vi "Main.vi"() -> ()   [LabVIEW 2020]
uses:
  <vilib>/userDefined/High Color/IMAQdx.ctl
  <vilib>/vision/Image Controls.llb/IMAQ Image.ctl
  <vilib>/DAQmx/read.llb/DAQmx Read (Analog Wfm 1Chan NSamp).vi
  <vilib>/Utility/error.llb/Error Cluster From Error Code.vi
  <vilib>/DAQmx/miscellaneous.llb/DAQmx Fill In Error Info.vi
  <vilib>/ErrorRing/Error Ring.xnode
  SuportVI2/Message Queue/Message Queue.lvlib
  SuportVI2/User Event - Stop/User Event - Stop.lvlib
  <vilib>/vision/driver/NI_Vision_Acquisition_Software.lvlib
panel:
  in  "Is start 2":bool=TRUE
  in  "Data":string="000001"
  in  "Is start":bool
  out "Waveform Graph":waveform(dbl)(graph)
  in  "Aquire Configuration":T1
  in  "Generator Configuration":T1
  out "Image":T2(plugin-control)
  in  "Camera Config":cluster{"Camera Select":T3}={"Camera Select"="cam0"}
  in  "Exit":bool
  in  "Stop Camera":bool
  in  "Start":bool
  out "Status Line":string
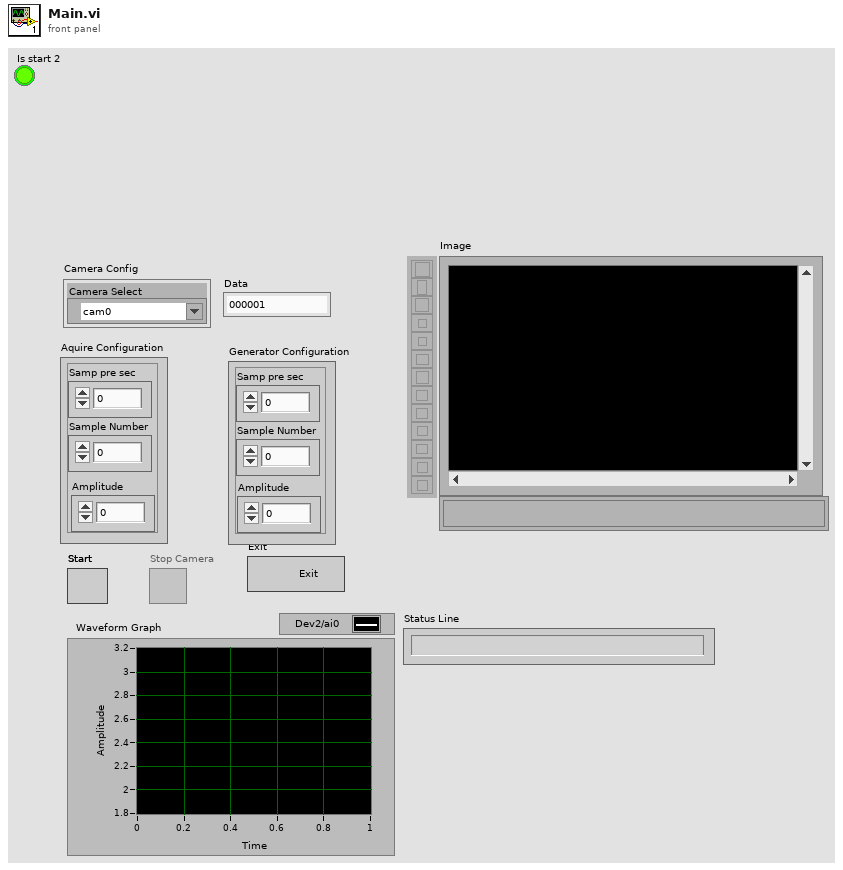
[diagram p1: front panel]
types:
  T1 = cluster{"Sample Number":dbl, "Samp pre sec":i32, "Amplitude":dbl}
  T2 = typedef "IMAQ Image.ctl" = refnum<image>
  T3 = typedef "IMAQdx.ctl" = refnum<k21>
  T4 = cluster{"configuration file path out":path, "DAQmx Task":refnum<k21>, "DAQmx Chanel":cluster{"SampClk.Rate":dbl, "SampQuant.SampPerChan":i32, "Amplitude 2":dbl}}
  T5 = cluster{"DAQmx Task":refnum<k21>, "DB Data":dbl[][], "DAQmx Chanel":cluster{"SampClk.Rate":dbl, "SampQuant.SampPerChan":i32, "Amplitude":dbl}}
  T6 = cluster{"Image":cluster{"Image original":T2, "Image copy":T2, "Image Out":T2}, "Session Config":cluster{"Session":T3}, "Data":string}
  T7 = cluster{"Start Camera":refnum<vi>, "Stop Camera":refnum<vi>, "Exit":refnum<vi>, "Camera Conf":refnum<vi>, "Status Line":refnum<vi>, "Status Line Text":string, "Camera Select":refnum<vi>, "Start Acquire":refnum<vi>, "Stop Acquire":refnum<vi>, "Start SinusGen":refnum<vi>, "Stop SinusGen":refnum<vi>, "Generator Configuration":refnum<vi>, "Aquire Configuration":refnum<vi>}
  T8 = cluster{"UI":refnum<queue>, "Camera":refnum<queue>, "Acquire":refnum<queue>, "SinusGen":refnum<queue>}
  T9 = typedef "Image Type" = u32
  T10 = cluster{"SampClk.Rate":dbl, "SampQuant.SampPerChan":i32, dbl}
  T11 = cluster{"SampClk.Rate":dbl, "SampQuant.SampPerChan":i32, "Amplitude":dbl}
  T12 = cluster{"SampClk.Rate":dbl, "SampQuant.SampPerChan":i32, "Amplitude 2":dbl}
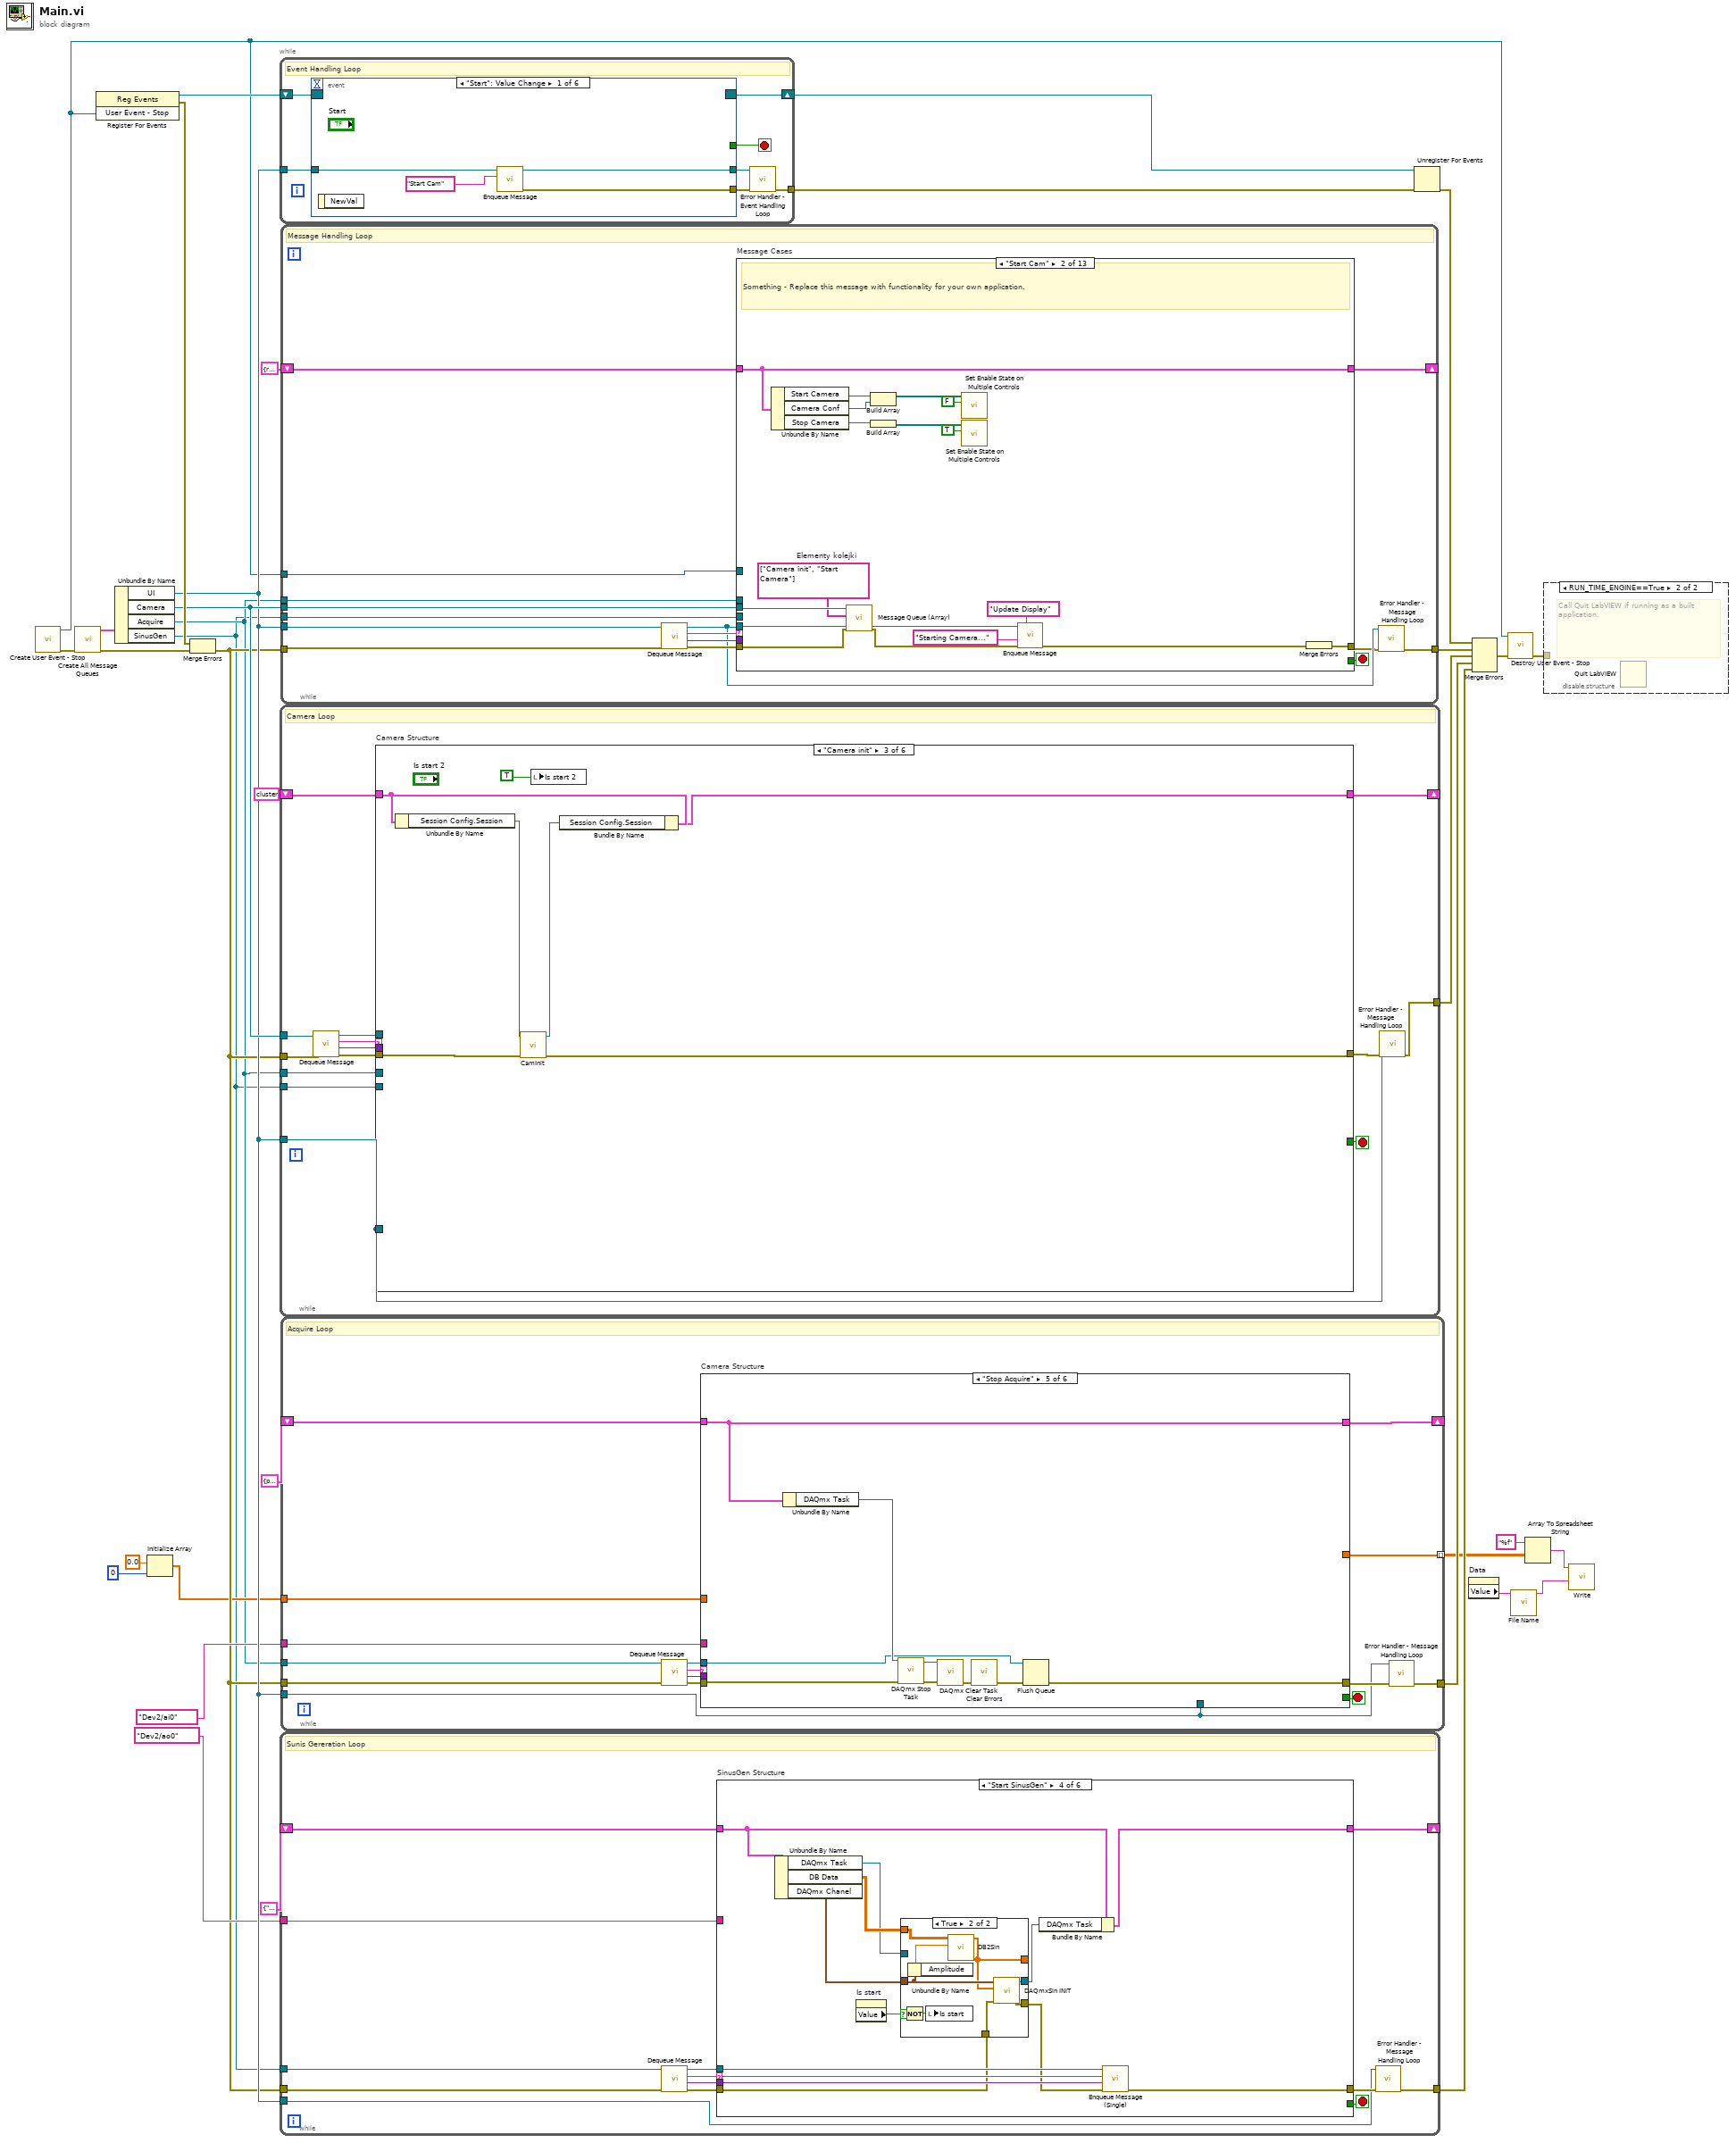
[diagram p0: block diagram]
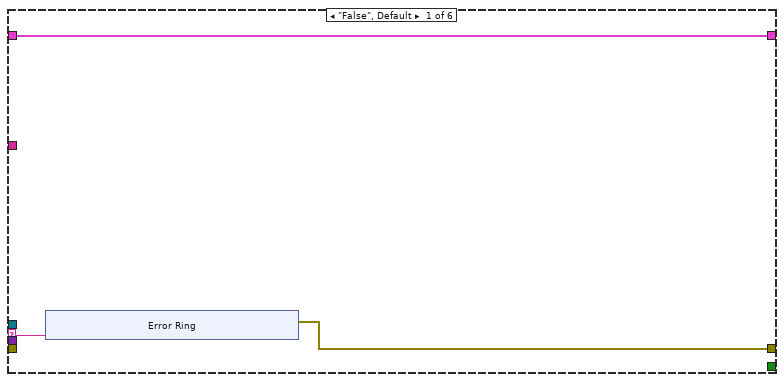
[diagram p2: hidden frame]
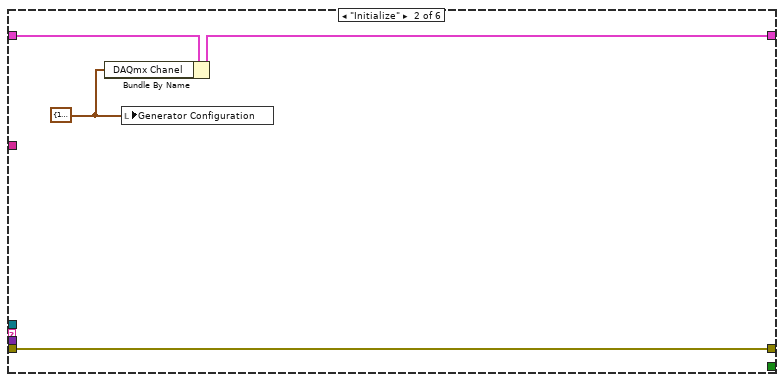
[diagram p3: hidden frame]
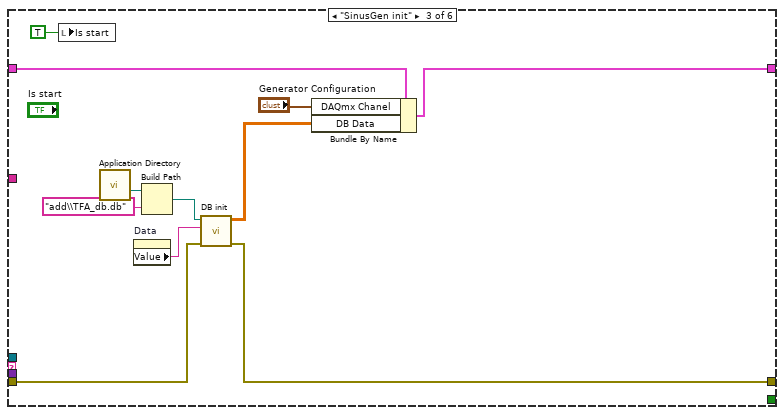
[diagram p4: hidden frame]
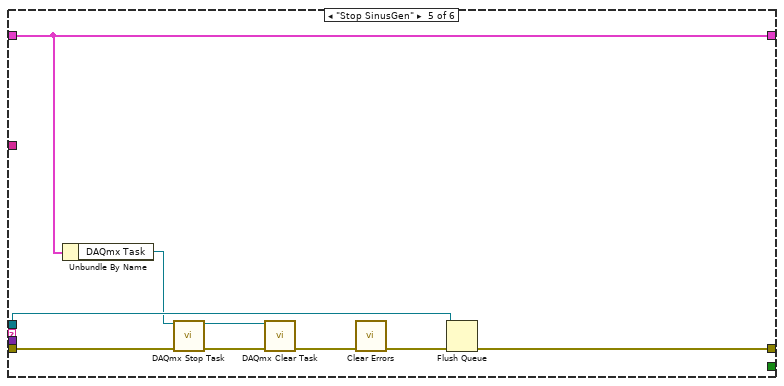
[diagram p6: hidden frame]
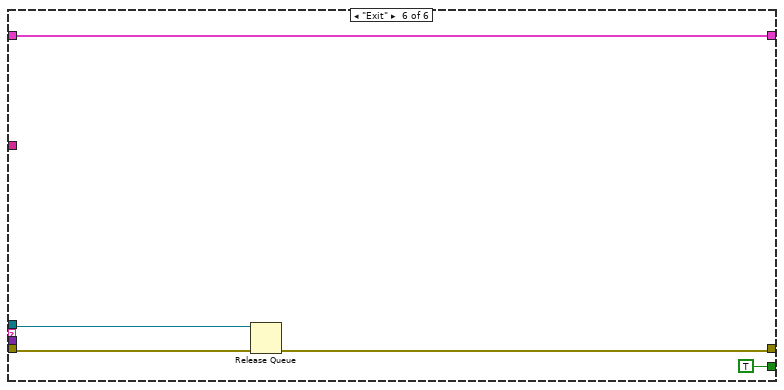
[diagram p7: hidden frame]
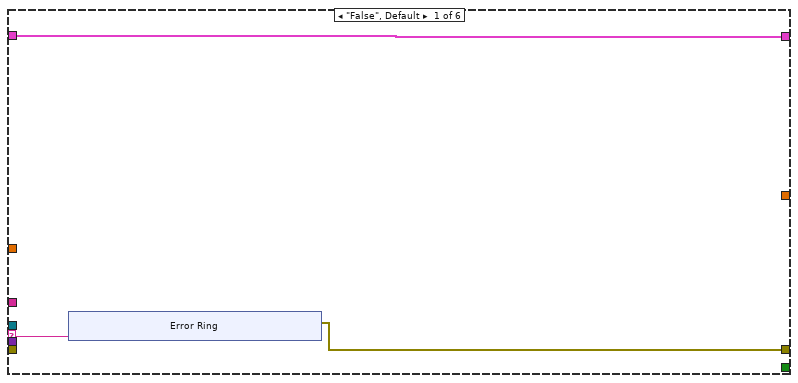
[diagram p8: hidden frame]
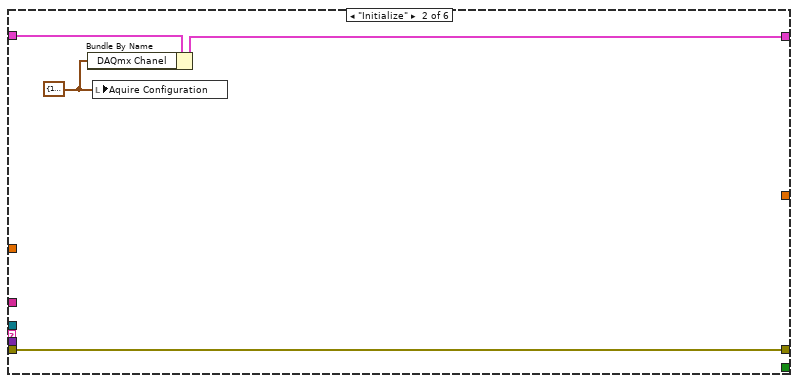
[diagram p9: hidden frame]
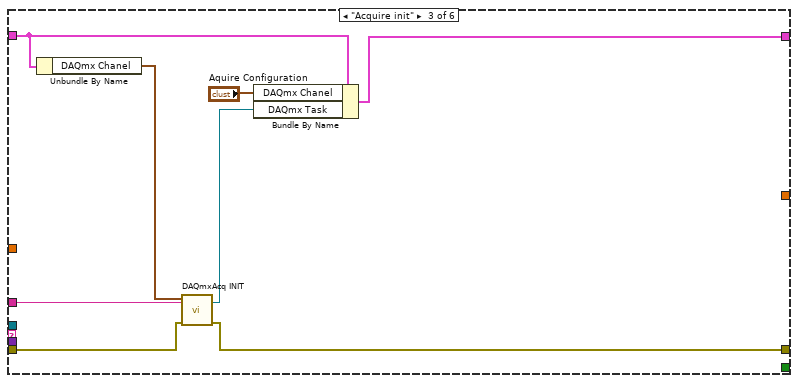
[diagram p10: hidden frame]
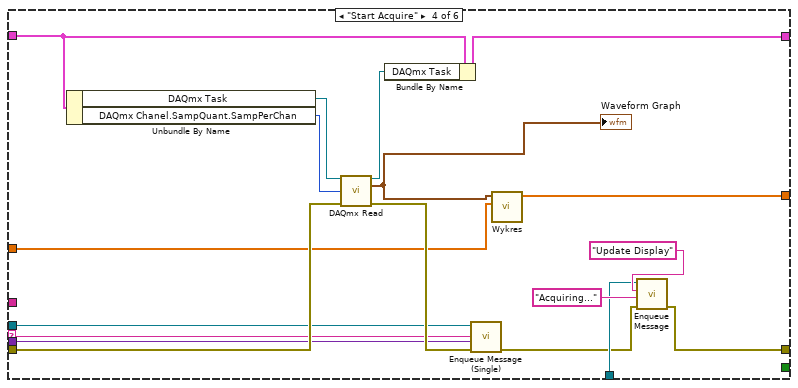
[diagram p11: hidden frame]
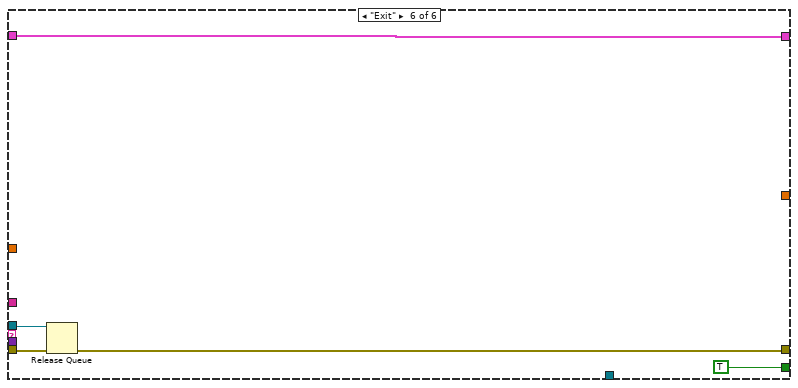
[diagram p12: hidden frame]
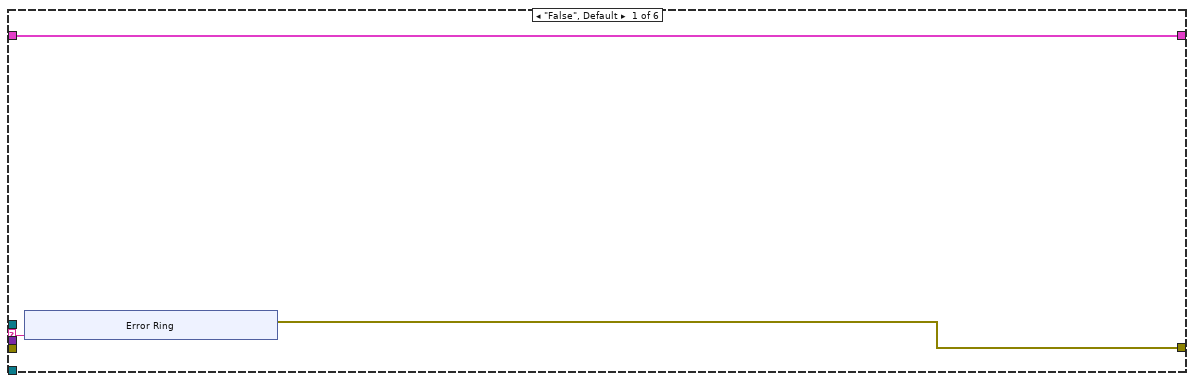
[diagram p13: hidden frame]
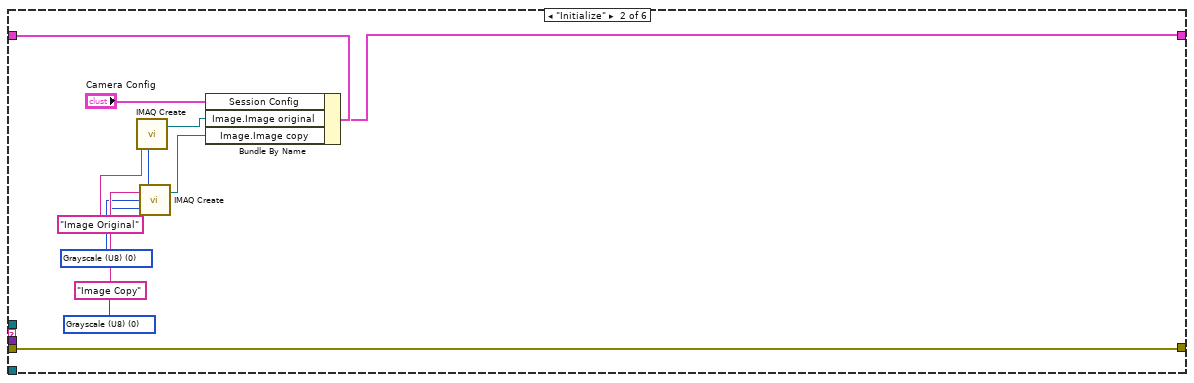
[diagram p14: hidden frame]
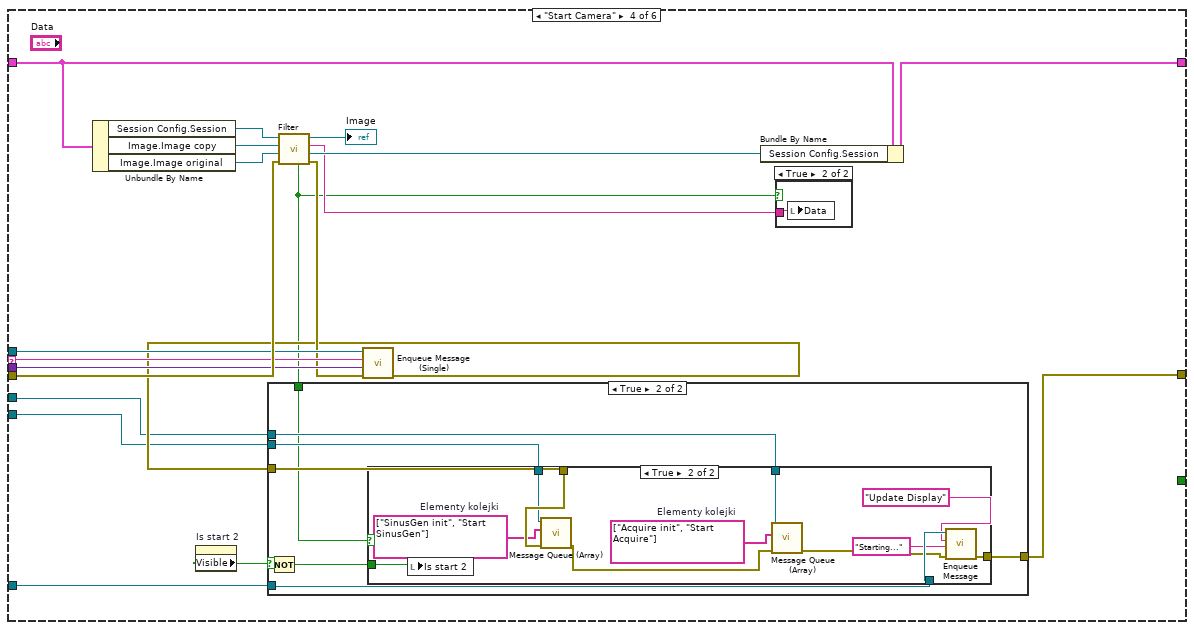
[diagram p15: hidden frame]
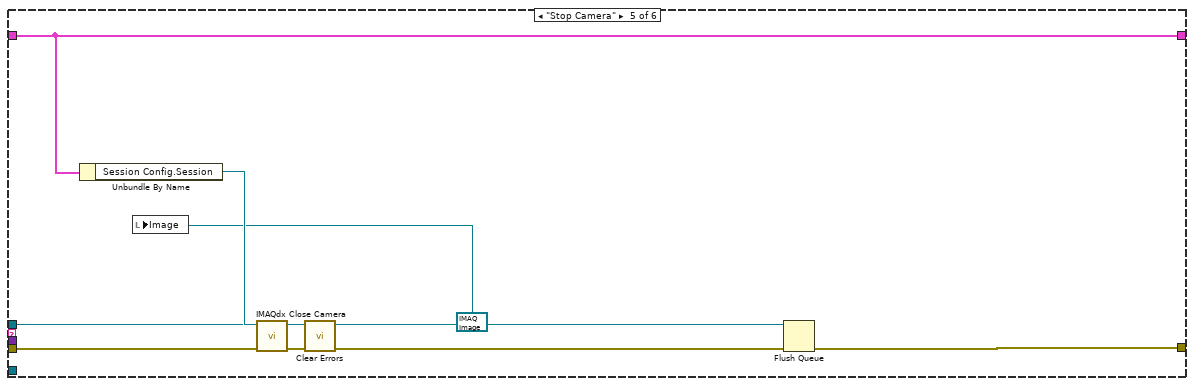
[diagram p19: hidden frame]
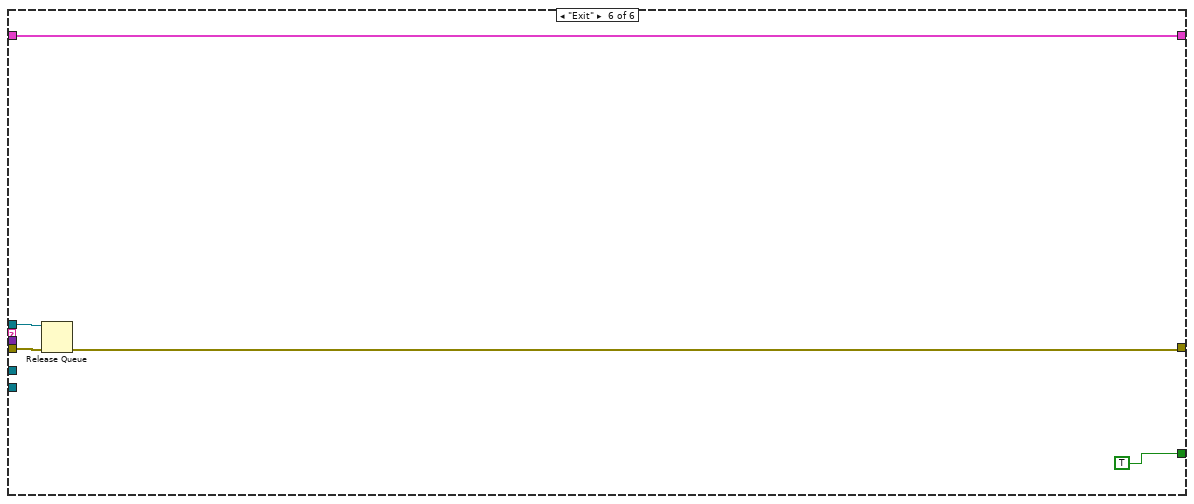
[diagram p20: hidden frame]
diagram:
  n1 = call "Create User Event - Stop.vi"() -> ("error out"=w32:errorcluster, "User Event - Stop"=w18:refnum<user-event>)  [unwired: 10 in]
  n2 = call "Create All Message Queues.vi"("error in (no error)"=w32) -> ("error out"=w34:errorcluster, "Message Queues out"=w22:T8)  [unwired: 9 in]
  n3 = register-events(w18) -> (reference out=w27:refnum<event-registration>, error out=w26:errorcluster)  [unwired: 2 in]
  n4 = Unbundle By Name(w22) -> ("UI"=w20:refnum<queue>, "Camera"=w21:refnum<queue>, "Acquire"=w2:refnum<queue>, "SinusGen"=w1:refnum<queue>)
  n5 = Initialize Array(0.0 ("element"), 0 ("dimension size")) -> (w6:dbl[])
  n6 = Merge Errors(w26, w34) -> (w14:errorcluster)
  n7 = while {
    tunnel: w20 -> [w41]
    shift-right: [w39] -> w30
    shift-left: w27 -> [w40]
    tunnel: [w35] -> w28
    stop <- w37 stop-if-true
    # "Event Handling Loop"
    n8 = event shown="[0] \"Start\": Value Change" {
      selector: w40 -> [_ _ _ _ _ _]
      dyn-events: [_ _ _ _ _ _] -> w39
      timeout: _ -> [_ _ _ _ _ _]
      tunnel: [_ _ _ _ _ TRUE ("Discard?")] -> w37
      tunnel: w41 -> [w45 w49 w54 w56 w61 w64]
      tunnel: [w42 w46 w53 _ w60 _] -> w38
      tunnel: [w44 w48 w52 w56 w59 w64] -> w36
      event "Start": Value Change {
        n9 = event-data() -> ()  [unwired: 1 in, 1 out]
        n10 = call-poly "Enqueue Message.vi"("Message"="Start Cam", "Message Queue"=w45) -> ("error out"=w42:errorcluster, "dup Message Queue"=w44:refnum<queue>)  [unwired: 8 in]
      }
      event "Stop Camera": Value Change {
        n11 = event-data() -> ()  [unwired: 1 in, 1 out]
        n12 = call-poly "Enqueue Message.vi"("Message"="Stop Cam", "Message Queue"=w49) -> ("error out"=w46:errorcluster, "dup Message Queue"=w48:refnum<queue>)  [unwired: 8 in]
      }
      event Panel Close? {
        # "Send the 'Confirm Quit' message if the user closes the panel of the VI. Discard the event so the 'Confirm Quit' message has a chance to run."
        n13 = event-data() -> ()  [unwired: 1 in, 1 out]
        n14 = call-poly "Enqueue Message.vi"("Priority Message? (F)"=TRUE, "Message"="Confirm Quit", "Message Queue"=w54) -> ("error out"=w53:errorcluster, "dup Message Queue"=w52:refnum<queue>)  [unwired: 7 in]
        n15 = event-data("Discard?"=TRUE) -> ()  [unwired: 1 in, 1 out]
      }
      event Application Instance Close {
        # "#CodeRecommended - When a project closes, all VIs within that project are aborted and leave memory. However, any code placed in this event frame is guaranteed to run to completion, so add any cleanup code that absolutely must happen here."
        n16 = event-data() -> ()  [unwired: 1 in, 1 out]
      }
      event "Exit": Value Change {
        n17 = event-data() -> ()  [unwired: 1 in, 1 out]
        n18 = call-poly "Enqueue Message.vi"("Priority Message? (F)"=TRUE, "Message"="Exit", "Message Queue"=w61) -> ("error out"=w60:errorcluster, "dup Message Queue"=w59:refnum<queue>)  [unwired: 7 in]
      }
      event User Event {
        # "The Message Handling Loop processed an \"Exit\" message, which fired this event to stop the Event Handling Loop."
        n19 = event-data() -> ()  [unwired: 1 in, 1 out]
        n20 = local write "Status Line"("Exiting application" ("VI Stopped")) -> ()
      }
    }
    n21 = call "Error Handler - Event Handling Loop.vi"("error in (no error)"=w38, "Message Queue"=w36) -> ("dup error in"=w35:errorcluster)  [unwired: 8 in, 1 out]
  }
  n22 = while {
    shift-right: [w71] -> _
    shift-left: T6 {"Image"={"Image original"=refnum, "Image copy"=refnum, "Image Out"=refnum}, "Session Config"={"Session"=""}, "Data"=""} ("Camera conf Cluster") -> [w74]
    tunnel: [w78] -> w24
    tunnel: w14 -> [w77]
    tunnel: w20 -> [w65]
    tunnel: w21 -> [w73]
    tunnel: w2 -> [w67]
    tunnel: w1 -> [w66]
    stop <- w69 stop-if-true
    # "Camera Loop"
    n23 = call "Dequeue Message.vi"("error in (no error)"=w77, "Message Queue"=w73) -> ("error out"=w76:errorcluster, "Message Data"=w70:variant, "Message"=w68:string, "dup Message Queue"=w72:refnum<queue>)  [unwired: 6 in]
    n24 = case "Camera Structure" shown="\"Camera init\"" w68 {
      selector: w68 -> [w79 _ _ w117 _ _]
      tunnel: [w81 w98 w102 w109 w151 w159] -> w75
      tunnel: w76 -> [_ w98 w103 w125 w156 w158]
      tunnel: w74 -> [w80 w96 w101 w121 w155 w161]
      tunnel: w72 -> [_ _ _ w118 w150 w160]
      tunnel: [w80 w95 w100 w119 w155 w161] -> w71
      tunnel: w70 -> [_ _ _ w116 _ _]
      tunnel: [_ _ _ _ _ TRUE] -> w69
      tunnel: w67 -> [_ _ _ w106 _ _]
      tunnel: w66 -> [_ _ _ w110 _ _]
      tunnel: w65 -> [_ _ _ w112 _ _]
      frame "False", Default {
        n25 = xnode "Error Ring"("parameter 0"=w79) -> ("error out"=w81:errorcluster)
      }
      frame "Initialize" {
        w90 = T9 0 items=["Grayscale (U8)", "Grayscale (I16)", "Grayscale (SGL)", "Complex (CSG)", "RGB (U32)", "HSL (U32)", "RGB (U64)", "Grayscale (U16)"] ("Image Type")
        w93 = T9 0 items=["Grayscale (U8)", "Grayscale (I16)", "Grayscale (SGL)", "Complex (CSG)", "RGB (U32)", "HSL (U32)", "RGB (U64)", "Grayscale (U16)"] ("Image Type")
        n26 = call "IMAQ Create"("Image Name"="Image Original", "Image Type"=w90) -> ("New Image"=w89:T2)  [unwired: 3 in, 1 out]
        n27 = call "IMAQ Create"("Image Name"="Image Copy", "Image Type"=w93) -> ("New Image"=w92:T2)  [unwired: 3 in, 1 out]
        n28 = Bundle By Name(cluster=w96, "Session Config"="Camera Config", "Image.Image original"=w89, "Image.Image copy"=w92) -> (w95:T6)
      }
      frame "Camera init" {
        n29 = Unbundle By Name(w101) -> ("Session Config.Session"=w105:T3)
        n30 = call "CamInit.vi"("error in (no error)"=w103, "Refnum in"=w105) -> ("error out"=w102:errorcluster, "Refnum out"=w104:T3)  [unwired: 8 in]
        n31 = local write "Is start 2"(TRUE ("Is start 2")) -> ()
        n32 = Bundle By Name(cluster=w101, "Session Config.Session"=w104) -> (w100:T6)
      }
      frame "Start Camera" {
        n33 = Unbundle By Name(w121) -> ("Session Config.Session"=w124:T3, "Image.Image copy"=w123:T2, "Image.Image original"=w122:T2)
        n34 = property on="Is start 2" class="Bool (strict)"() -> ("Visible"=w107:bool)  [unwired: 2 in, 2 out]
        n35 = call "Filter.vi"("error in"=w125, "Image original"=w122, "Image copy"=w123, "Session Config"=w124) -> ("error out"=w115:errorcluster, "Session Out"=w120:T3, "Data"=w113:string, "Image Out"=→"Image":T2, "Found?"=w108:bool)  [unwired: 3 in]
        n36 = call "Enqueue Message (Single).vi"("error in (no error)"=w115, "Message Data"=w116, "Message"=w117, "Message Queue"=w118) -> ("error out"=w111:errorcluster)  [unwired: 6 in, 1 out]
        n37 = case shown="True" w107 {
          selector: w107 -> [_ w128]
          tunnel: w112 -> [_ w134]
          tunnel: w106 -> [_ w133]
          tunnel: w111 -> [w126 w132]
          tunnel: w110 -> [_ w131]
          tunnel: [w126 w130] -> w109
          tunnel: w108 -> [_ w129]
          frame False {
          }
          frame True {
            n38 = Not(x=w128) -> (.not. x?=w127:bool)
            n39 = case shown="True" w129 {
              tunnel: w134 -> [_ w147]
              tunnel: w133 -> [_ w146]
              tunnel: w132 -> [w135 w145]
              tunnel: w131 -> [_ w144]
              tunnel: [w135 w143] -> w130
              tunnel: w127 -> [_ w136]
              frame False {
              }
              frame True {
                w137 = string[] ["Acquire init", "Start Acquire"]  # Elementy kolejki
                w138 = string[] ["SinusGen init", "Start SinusGen"]  # Elementy kolejki
                n40 = local write "Is start 2"(w136) -> ()
                n41 = call "Message Queue (Array).vi"("error in (no error)"=w145, "Message Array"=w138, "Message Queue"=w144) -> ("error out"=w139:errorcluster)  [unwired: 7 in, 1 out]
                n42 = call "Message Queue (Array).vi"("error in (no error)"=w139, "Message Array"=w137, "Message Queue"=w146) -> ("error out"=w142:errorcluster)  [unwired: 7 in, 1 out]
                n43 = call-poly "Enqueue Message.vi"("error in (no error)"=w142, "Message Data"="Starting..." ("\"Do Something\" button pressed"), "Message"="Update Display", "Message Queue"=w147) -> ("error out"=w143:errorcluster)  [unwired: 6 in, 1 out]
              }
            }
          }
        }
        n44 = Bundle By Name(cluster=w121, "Session Config.Session"=w120) -> (w119:T6)
        n45 = case shown="True" w108 {
          tunnel: w113 -> [_ w148]
          frame False {
          }
          frame True {
            n46 = local write "Data"(w148) -> ()
          }
        }
      }
      frame "Stop Camera" {
        n47 = Unbundle By Name(w155) -> ("Session Config.Session"=w154:T3)
        n48 = local write "Image"(T2 refnum ("Image")) -> ()
        n49 = call <vilib>:"IMAQdx Close Camera.vi"("error in"=w156, "Session In"=w154) -> ("error out"=w152:errorcluster)  [unwired: 9 in]
        n50 = call <vilib>:"Clear Errors.vi"("error in (no error)"=w152) -> ("error out"=w153:errorcluster)  [unwired: 5 in, 1 out]
        n51 = Flush Queue(queue=w150, error in (no error)=w153) -> (error out=w151:errorcluster)  [unwired: 2 out]
      }
      frame "Exit" {
        n52 = Release Queue(queue=w160, error in (no error)=w158) -> (error out=w159:errorcluster)  [unwired: 1 in, 2 out]
      }
    }
    n53 = call "Error Handler - Message Handling Loop.vi"("error in (no error)"=w75, "Message Queue"=w65) -> ("dup error in"=w78:errorcluster)  [unwired: 8 in, 1 out]
  }
  n54 = while {
    tunnel: w20 -> [w162]
    tunnel: w1 -> [w174]
    tunnel: tag "Dev2/ao0" ("physical channels") -> [w173]
    tunnel: w14 -> [w167]
    tunnel: [w163] -> w13
    shift-right: [w166] -> _
    shift-left: T5 {"DAQmx Task"="", "DB Data"=[[0.0]], "DAQmx Chanel"={"SampClk.Rate"=0.0, "SampQuant.SampPerChan"=0, "Amplitude"=0.0}} -> [w165]
    stop <- w164 stop-if-true
    # "Sunis Gereration Loop"
    n55 = call "Dequeue Message.vi"("error in (no error)"=w167, "Message Queue"=w174) -> ("error out"=w172:errorcluster, "Message Data"=w169:variant, "Message"=w168:string, "dup Message Queue"=w170:refnum<queue>)  [unwired: 6 in]
    n56 = case "SinusGen Structure" shown="\"Start SinusGen\"" w168 {
      selector: w168 -> [w176 _ _ w211 _ _]
      tunnel: [w177 w186 w192 w209 w231 w236] -> w171
      tunnel: w172 -> [_ w186 w197 w203 w225 w235]
      tunnel: w170 -> [_ _ _ w212 w230 w237]
      tunnel: w169 -> [_ _ _ w210 _ _]
      tunnel: [_ _ _ _ _ TRUE] -> w164
      tunnel: [w175 w187 w198 w207 w227 w233] -> w166
      tunnel: w165 -> [w175 w188 w199 w208 w227 w233]
      tunnel: w173 -> [_ _ _ _ _ _]
      frame "False", Default {
        n57 = xnode "Error Ring"("parameter 0"=w176) -> ("error out"=w177:errorcluster)
      }
      frame "Initialize" {
        w185 = T10 {"SampClk.Rate"=1000.0, "SampQuant.SampPerChan"=1000, 5.0} ("DAQmx Chanel")
        n58 = Bundle By Name(cluster=w188, "DAQmx Chanel"=w185) -> (w187:T5)
        n59 = local write "Generator Configuration"(w185) -> ()
      }
      frame "SinusGen init" {
        n60 = local write "Is start"(TRUE ("Boolean")) -> ()
        n61 = call <vilib>:"Application Directory.vi"() -> ("Application Directory"=w196:path)
        n62 = property on="Data" class="Str"() -> ("Value"=w189:string)  [unwired: 2 in, 2 out]
        n63 = Build Path(base path=w196, name or relative path="add\\TFA_db.db") -> (appended path=w194:path)
        n64 = call "DB init.vi"("error in (no error)"=w197, "ID"=w189, "DB path"=w194) -> ("error out"=w192:errorcluster, "DB Data"=w191:dbl[][])  [unwired: 6 in, 1 out]
        n65 = Bundle By Name(cluster=w199, "DAQmx Chanel"="Generator Configuration", "DB Data"=w191) -> (w198:T5)
      }
      frame "Start SinusGen" {
        n66 = Unbundle By Name(w208) -> ("DAQmx Task"=w201:refnum<k21>, "DB Data"=w206:dbl[][], "DAQmx Chanel"=w205:T11)
        n67 = property on="Is start" class="Bool (strict)"() -> ("Value"=w200:bool)  [unwired: 2 in, 2 out]
        n68 = case shown="True" w200 {
          selector: w200 -> [_ w219]
          tunnel: w206 -> [_ w223]
          tunnel: w205 -> [_ w217]
          tunnel: [w213 w222] -> w204
          tunnel: w203 -> [w214 w221]
          tunnel: [w214 w220] -> w202
          tunnel: w201 -> [w213 _]
          tunnel: [_ w215] -> _
          frame False {
          }
          frame True {
            n69 = Not(x=w219) -> (.not. x?=w218:bool)
            n70 = Unbundle By Name(w217) -> ("Amplitude"=w216:dbl)
            n71 = local write "Is start"(w218) -> ()
            n72 = call "DB2Sin.vi"("amplitude"=w216, "DB Data"=w223) -> ("sine wave"=w215:dbl[])  [unwired: 9 in]
            n73 = call "DAQmxSin INIT.vi"("error in"=w221, "sine wave"=w215, "DAQmxChannel"=w217) -> ("error out"=w220:errorcluster, "task out"=w222:refnum<k21>)  [unwired: 7 in]
          }
        }
        n74 = Bundle By Name(cluster=w208, "DAQmx Task"=w204) -> (w207:T5)
        n75 = call "Enqueue Message (Single).vi"("error in (no error)"=w202, "Message Data"=w210, "Message"=w211, "Message Queue"=w212) -> ("error out"=w209:errorcluster)  [unwired: 6 in, 1 out]
      }
      frame "Stop SinusGen" {
        n76 = Unbundle By Name(w227) -> ("DAQmx Task"=w226:refnum<k21>)
        n77 = call <vilib>:"DAQmx Stop Task.vi"("task/channels in"=w226, "error in"=w225) -> ("task out"=w229:refnum<k21>, "error out"=w228:errorcluster)  [unwired: 12 in]
        n78 = call <vilib>:"DAQmx Clear Task.vi"("task in"=w229, "error in"=w228) -> ("error out"=w224:errorcluster)  [unwired: 13 in]
        n79 = call <vilib>:"Clear Errors.vi"("error in (no error)"=w224) -> ("error out"=w232:errorcluster)  [unwired: 5 in, 1 out]
        n80 = Flush Queue(queue=w230, error in (no error)=w232) -> (error out=w231:errorcluster)  [unwired: 2 out]
      }
      frame "Exit" {
        n81 = Release Queue(queue=w237, error in (no error)=w235) -> (error out=w236:errorcluster)  [unwired: 1 in, 2 out]
      }
    }
    n82 = call "Error Handler - Message Handling Loop.vi"("error in (no error)"=w171, "Message Queue"=w162) -> ("dup error in"=w163:errorcluster)  [unwired: 8 in, 1 out]
  }
  n83 = while {
    tunnel: w20 -> [w245]
    shift-right: [w251] -> _
    shift-left: T7 {"Start Camera"=refnum, "Stop Camera"=refnum, "Exit"=refnum, "Camera Conf"=refnum, "Status Line"=refnum, "Status Line Text"="", "Camera Select"=refnum, "Start Acquire"=refnum, "Stop Acquire"=refnum, "Start SinusGen"=refnum, "Stop SinusGen"=refnum, "Generator Configuration"=refnum, "Aquire Configuration"=refnum} -> [w252]
    tunnel: w18 -> [w249]
    tunnel: w14 -> [w238]
    tunnel: [w243] -> w33
    tunnel: w21 -> [w241]
    tunnel: w2 -> [w240]
    tunnel: w1 -> [w239]
    stop <- w250 stop-if-true
    # "Message Handling Loop"
    n84 = call "Dequeue Message.vi"("error in (no error)"=w238, "Message Queue"=w245) -> ("error out"=w248:errorcluster, "Message Data"=w246:variant, "Message"=w247:string, "dup Message Queue"=w244:refnum<queue>)  [unwired: 6 in]
    n85 = case "Message Cases" shown="\"Start Cam\"" w247 {
      selector: w247 -> [_ _ _ _ _ _ _ _ _ _ _ _ w404]
      tunnel: w244 -> [w264 w283 w296 w309 w329 w347 w365 _ _ w384 _ w403 _]
      tunnel: w248 -> [w269 w280 w294 w307 w326 w344 w362 w372 w381 w388 w391 w393 _]
      tunnel: [w270 w287 w300 w313 w331 w349 w367 w373 w375 w386 w389 w400 w405] -> w242
      tunnel: w252 -> [w268 w278 w292 w305 w314 w333 w351 w374 w380 w387 w390 w397 w406]
      tunnel: [w267 w278 w292 w305 w314 w333 w351 w374 w380 w387 w390 w397 w406] -> w251
      tunnel: [_ _ _ _ _ _ _ _ _ _ _ TRUE _] -> w250
      tunnel: w246 -> [_ _ _ _ _ _ _ w371 w379 _ _ _ _]
      tunnel: w249 -> [_ _ _ _ _ _ _ _ _ _ _ w399 _]
      tunnel: w241 -> [_ w282 _ _ w324 _ _ _ _ _ _ w395 _]
      tunnel: w240 -> [_ _ _ w301 _ _ w350 _ _ _ _ w396 _]
      tunnel: w239 -> [_ _ w288 _ _ w332 _ _ _ _ _ w394 _]
      frame "Initialize" {
        w263 = "Initialization Completed" ("Initial Message")
        # "Initialize - All initialization work should take place in this message, since other loops can potentially enqueue messages that execute immediately after this one."
        n86 = control-ref of="Start"() -> (w255:refnum<vi>)
        n87 = control-ref of="Stop Camera"() -> (w260:refnum<vi>)
        n88 = control-ref of="Exit"() -> (w257:refnum<vi>)
        n89 = control-ref of="Camera Config"() -> (w256:refnum<vi>)
        n90 = control-ref of="Generator Configuration"() -> (w253:refnum<vi>)
        n91 = control-ref of="Aquire Configuration"() -> (w254:refnum<vi>)
        n92 = control-ref of="Status Line"() -> (w266:refnum<vi>)
        n93 = Bundle By Name(cluster=w268, "Start Camera"=w255, "Stop Camera"=w260, "Status Line"=w266, "Exit"=w257, "Status Line Text"=w263, "Camera Select"=w256, "Generator Configuration"=w253, "Aquire Configuration"=w254) -> (w267:T7)
        n94 = call-poly "Enqueue Message.vi"("error in (no error)"=w269, "Message Data"=w263, "Message"="Update Display", "Message Queue"=w264) -> ("error out"=w270:errorcluster)  [unwired: 6 in, 1 out]
        n95 = Build Array(w260) -> (w261:refnum<vi>[])
        n96 = call "Set Enable State on Multiple Controls.vi"("Enable?"=FALSE, "Controls"=w261) -> ()  [unwired: 10 in]
        n97 = Build Array(w255, w257, w256, w254, w253) -> (w259:refnum<vi>[])
        n98 = call "Set Enable State on Multiple Controls.vi"("Enable?"=TRUE, "Controls"=w259) -> ()  [unwired: 10 in]
      }
      frame "Start Cam" {
        w281 = string[] ["Camera init", "Start Camera"]  # Elementy kolejki
        # "Something - Replace this message with functionality for your own application."
        n99 = Unbundle By Name(w278) -> ("Start Camera"=w272:refnum<vi>, "Camera Conf"=w273:refnum<vi>, "Stop Camera"=w274:refnum<vi>)
        n100 = call "Message Queue (Array).vi"("error in (no error)"=w280, "Message Array"=w281, "Message Queue"=w282) -> ("error out"=w279:errorcluster)  [unwired: 7 in, 1 out]
        n101 = Build Array(w272, w273) -> (w277:refnum<vi>[])
        n102 = Build Array(w274) -> (w276:refnum<vi>[])
        n103 = call "Set Enable State on Multiple Controls.vi"("Enable?"=FALSE, "Controls"=w277) -> ()  [unwired: 10 in]
        n104 = call "Set Enable State on Multiple Controls.vi"("Enable?"=TRUE, "Controls"=w276) -> ()  [unwired: 10 in]
        n105 = call-poly "Enqueue Message.vi"("error in (no error)"=w279, "Message Data"="Starting Camera..." ("\"Do Something\" button pressed"), "Message"="Update Display", "Message Queue"=w283) -> ("error out"=w286:errorcluster)  [unwired: 6 in, 1 out]
        n106 = Merge Errors(w286) -> (w287:errorcluster)
      }
      frame "Start SinGen" {
        w295 = string[] ["SinusGen init", "Start SinusGen"]  # Elementy kolejki
        # "Something - Replace this message with functionality for your own application."
        n107 = Unbundle By Name(w292) -> ("Generator Configuration"=w289:refnum<vi>)
        n108 = call "Message Queue (Array).vi"("error in (no error)"=w294, "Message Array"=w295, "Message Queue"=w288) -> ("error out"=w293:errorcluster)  [unwired: 7 in, 1 out]
        n109 = Build Array(w289) -> (w291:refnum<vi>[])
        n110 = call "Set Enable State on Multiple Controls.vi"("Enable?"=FALSE, "Controls"=w291) -> ()  [unwired: 10 in]
        n111 = call-poly "Enqueue Message.vi"("error in (no error)"=w293, "Message Data"="Starting SinusGen..." ("\"Do Something\" button pressed"), "Message"="Update Display", "Message Queue"=w296) -> ("error out"=w299:errorcluster)  [unwired: 6 in, 1 out]
        n112 = Merge Errors(w299) -> (w300:errorcluster)
      }
      frame "Start Acq" {
        w308 = string[] ["Acquire init", "Start Acquire"]  # Elementy kolejki
        # "Something - Replace this message with functionality for your own application."
        n113 = Unbundle By Name(w305) -> ("Aquire Configuration"=w302:refnum<vi>)
        n114 = call "Message Queue (Array).vi"("error in (no error)"=w307, "Message Array"=w308, "Message Queue"=w301) -> ("error out"=w306:errorcluster)  [unwired: 7 in, 1 out]
        n115 = Build Array(w302) -> (w304:refnum<vi>[])
        n116 = call "Set Enable State on Multiple Controls.vi"("Enable?"=FALSE, "Controls"=w304) -> ()  [unwired: 10 in]
        n117 = call-poly "Enqueue Message.vi"("error in (no error)"=w306, "Message Data"="Starting Acquire..." ("\"Do Something\" button pressed"), "Message"="Update Display", "Message Queue"=w309) -> ("error out"=w312:errorcluster)  [unwired: 6 in, 1 out]
        n118 = Merge Errors(w312) -> (w313:errorcluster)
      }
      frame "Stop Cam" {
        # "Something Else - Replace this message with functionality for your own application."
        n119 = Unbundle By Name(w314) -> ("Start Camera"=w316:refnum<vi>, "Camera Conf"=w317:refnum<vi>, "Stop Camera"=w318:refnum<vi>)
        n120 = call-poly "Enqueue Message.vi"("Priority Message? (F)"=TRUE, "error in (no error)"=w326, "Message"="Stop Camera", "Message Queue"=w324) -> ("error out"=w325:errorcluster)  [unwired: 6 in, 1 out]
        n121 = Build Array(w316, w317) -> (w321:refnum<vi>[])
        n122 = Build Array(w318) -> (w320:refnum<vi>[])
        n123 = call-poly "Enqueue Message.vi"("error in (no error)"=w325, "Message Data"="Camera Stopped" ("\"Do Something Else\" button pressed"), "Message"="Update Display", "Message Queue"=w329) -> ("error out"=w330:errorcluster)  [unwired: 6 in, 1 out]
        n124 = call "Set Enable State on Multiple Controls.vi"("Enable?"=TRUE, "Controls"=w321) -> ()  [unwired: 10 in]
        n125 = call "Set Enable State on Multiple Controls.vi"("Enable?"=FALSE, "Controls"=w320) -> ()  [unwired: 10 in]
        n126 = Merge Errors(w330) -> (w331:errorcluster)
      }
      frame "Stop SinGen" {
        # "Something Else - Replace this message with functionality for your own application."
        n127 = Unbundle By Name(w333) -> ("Start SinusGen"=w335:refnum<vi>, "Generator Configuration"=w336:refnum<vi>, "Stop SinusGen"=w337:refnum<vi>)
        n128 = call-poly "Enqueue Message.vi"("Priority Message? (F)"=TRUE, "error in (no error)"=w344, "Message"="Stop SinusGen", "Message Queue"=w332) -> ("error out"=w343:errorcluster)  [unwired: 6 in, 1 out]
        n129 = Build Array(w335, w336) -> (w340:refnum<vi>[])
        n130 = Build Array(w337) -> (w339:refnum<vi>[])
        n131 = call "Set Enable State on Multiple Controls.vi"("Enable?"=TRUE, "Controls"=w340) -> ()  [unwired: 10 in]
        n132 = call "Set Enable State on Multiple Controls.vi"("Enable?"=FALSE, "Controls"=w339) -> ()  [unwired: 10 in]
        n133 = call-poly "Enqueue Message.vi"("error in (no error)"=w343, "Message Data"="SinusGen Stopped" ("\"Do Something Else\" button pressed"), "Message"="Update Display", "Message Queue"=w347) -> ("error out"=w348:errorcluster)  [unwired: 6 in, 1 out]
        n134 = Merge Errors(w348) -> (w349:errorcluster)
      }
      frame "Stop Acq" {
        # "Something Else - Replace this message with functionality for your own application."
        n135 = Unbundle By Name(w351) -> ("Start Acquire"=w353:refnum<vi>, "Aquire Configuration"=w354:refnum<vi>, "Stop Acquire"=w355:refnum<vi>)
        n136 = call-poly "Enqueue Message.vi"("Priority Message? (F)"=TRUE, "error in (no error)"=w362, "Message"="Stop Acquire", "Message Queue"=w350) -> ("error out"=w361:errorcluster)  [unwired: 6 in, 1 out]
        n137 = Build Array(w353, w354) -> (w358:refnum<vi>[])
        n138 = Build Array(w355) -> (w357:refnum<vi>[])
        n139 = call "Set Enable State on Multiple Controls.vi"("Enable?"=TRUE, "Controls"=w358) -> ()  [unwired: 10 in]
        n140 = call "Set Enable State on Multiple Controls.vi"("Enable?"=FALSE, "Controls"=w357) -> ()  [unwired: 10 in]
        n141 = call-poly "Enqueue Message.vi"("error in (no error)"=w361, "Message Data"="Acquire Stopped" ("\"Do Something Else\" button pressed"), "Message"="Update Display", "Message Queue"=w365) -> ("error out"=w366:errorcluster)  [unwired: 6 in, 1 out]
        n142 = Merge Errors(w366) -> (w367:errorcluster)
      }
      frame "Update Display" {
        # "Update Display - Convert the message data to a string to display in the Data Display indicator."
        n143 = Variant To Data(error in=w372, type="", Variant=w371) -> (data=→"Status Line":string, error out=w369:errorcluster)
        n144 = Merge Errors(w369) -> (w373:errorcluster)
      }
      frame "Error" {
        # "Error - Display an error dialog. This message is sent by the \"Error Handler\" VIs at the end of other loops in this application."
        n145 = Variant To Data(error in=w381, type=errorcluster {"status"=FALSE, "code"=0, "source"=""} ("error constant"), Variant=w379) -> (data=w377:errorcluster, error out=w376:errorcluster)
        n146 = call <vilib>:"Simple Error Handler.vi"("error in (no error)"=w377) -> ()  [unwired: 4 in, 5 out]
        n147 = Merge Errors(w376) -> (w375:errorcluster)
      }
      frame "Confirm Quit" {
        # "Confirm Quit - Message that can confirm whether or not the user wants to exit the application."
        n148 = call-poly "Enqueue Message.vi"("Priority Message? (F)"=TRUE, "error in (no error)"=w388, "Message"="Exit", "Message Queue"=w384) -> ("error out"=w385:errorcluster)  [unwired: 6 in, 1 out]
        n149 = Merge Errors(w385) -> (w386:errorcluster)
      }
      frame "---Copy This Frame---" {
        # "Duplicate this frame when creating new messages.  Change this comment in the duplicated frame to describe this message."
        n150 = Merge Errors(w391) -> (w389:errorcluster)
      }
      frame "Exit" {
        # "Exit - Exit the application."
        n151 = call "Exit.vi"("error in"=w393, "Message Sin"=w394, "Message Acq"=w396, "Message Cam"=w395) -> ("error out"=w392:errorcluster)  [unwired: 7 in]
        n152 = call "Fire User Event - Stop.vi"("User Event - Stop"=w399) -> ("error out"=w398:errorcluster)  [unwired: 10 in]
        n153 = Release Queue(queue=w403, error in (no error)=w392) -> (error out=w401:errorcluster)  [unwired: 1 in, 2 out]
        n154 = Merge Errors(w398, w401) -> (w400:errorcluster)
      }
      frame Default {
        # "'Default' case only runs if there is a message that isn't defined in any of the other cases.  Output a programming error."
        n155 = xnode "Error Ring"("parameter 0"=w404) -> ("error out"=w405:errorcluster)
      }
    }
    n156 = call "Error Handler - Message Handling Loop.vi"("error in (no error)"=w242, "Message Queue"=w244) -> ("dup error in"=w243:errorcluster)  [unwired: 8 in, 1 out]
  }
  n157 = while {
    shift-right: [w420] -> _
    shift-left: T4 {"configuration file path out"=path "", "DAQmx Task"="", "DAQmx Chanel"={"SampClk.Rate"=0.0, "SampQuant.SampPerChan"=0, "Amplitude 2"=0.0}} -> [w419]
    tunnel: [w417] -> w17
    tunnel: w2 -> [w426]
    tunnel: w14 -> [w421]
    tunnel: w20 -> [w414]
    tunnel: tag "Dev2/ai0" ("physical channels") -> [w418]
    tunnel: [w416] -> w9 mode=indexing
    tunnel: w6 -> [w415]
    stop <- w423 stop-if-true
    # "Acquire Loop"
    n158 = call "Dequeue Message.vi"("error in (no error)"=w421, "Message Queue"=w426) -> ("error out"=w428:errorcluster, "Message Data"=w424:variant, "Message"=w422:string, "dup Message Queue"=w425:refnum<queue>)  [unwired: 6 in]
    n159 = case "Camera Structure" shown="\"Stop Acquire\"" w422 {
      selector: w422 -> [w430 _ _ w462 _ _]
      tunnel: [w431 w440 w443 w451 w472 w481] -> w427
      tunnel: w428 -> [_ w440 w446 w464 w471 w480]
      tunnel: w425 -> [_ _ _ w461 w469 w482]
      tunnel: w424 -> [_ _ _ w463 _ _]
      tunnel: [_ _ _ _ _ TRUE] -> w423
      tunnel: [w429 w441 w449 w466 w473 w478] -> w420
      tunnel: w419 -> [w429 w442 w450 w467 w473 w478]
      tunnel: w418 -> [_ _ w444 _ _ _]
      tunnel: [_ _ _ w458 _ _] -> w416
      tunnel: w415 -> [_ _ _ w457 _ _]
      tunnel: w414 -> [_ _ _ w453 _ _]
      frame "False", Default {
        n160 = xnode "Error Ring"("parameter 0"=w430) -> ("error out"=w431:errorcluster)
      }
      frame "Initialize" {
        w439 = T11 {"SampClk.Rate"=1000.0, "SampQuant.SampPerChan"=1000, "Amplitude"=5.0} ("DAQmx Chanel")
        n161 = Bundle By Name(cluster=w442, "DAQmx Chanel"=w439) -> (w441:T4)
        n162 = local write "Aquire Configuration"(w439) -> ()
      }
      frame "Acquire init" {
        n163 = Unbundle By Name(w450) -> ("DAQmx Chanel"=w447:T12)
        n164 = call "DAQmxAcq INIT.vi"("physical channels"=w444, "error in"=w446, "DAQmxChannel"=w447) -> ("error out"=w443:errorcluster, "task out"=w445:refnum<k21>)  [unwired: 7 in]
        n165 = Bundle By Name(cluster=w450, "DAQmx Chanel"="Aquire Configuration", "DAQmx Task"=w445) -> (w449:T4)
      }
      frame "Start Acquire" {
        n166 = Unbundle By Name(w467) -> ("DAQmx Task"=w460:refnum<k21>, "DAQmx Chanel.SampQuant.SampPerChan"=w465:i32)
        n167 = call-poly <vilib>:"DAQmx Read.vi"("task/channels in"=w460, "number of samples per channel"=w465, "error in"=w464) -> ("task out"=w459:refnum<k21>, "data"=w456:waveform(dbl), "error out"=w468:errorcluster)  [unwired: 10 in]
        "Waveform Graph" <- w456
        n168 = Bundle By Name(cluster=w467, "DAQmx Task"=w459) -> (w466:T4)
        n169 = call "Enqueue Message (Single).vi"("error in (no error)"=w468, "Message Data"=w463, "Message"=w462, "Message Queue"=w461) -> ("error out"=w452:errorcluster)  [unwired: 6 in, 1 out]
        n170 = call "Wykres.vi"("initialized array"=w457, "Y"=w456) -> ("output array"=w458:dbl[])  [unwired: 9 in]
        n171 = call-poly "Enqueue Message.vi"("error in (no error)"=w452, "Message Data"="Acquiring..." ("\"Do Something\" button pressed"), "Message"="Update Display", "Message Queue"=w453) -> ("error out"=w451:errorcluster)  [unwired: 6 in, 1 out]
      }
      frame "Stop Acquire" {
        n172 = Unbundle By Name(w473) -> ("DAQmx Task"=w470:refnum<k21>)
        n173 = call <vilib>:"DAQmx Stop Task.vi"("task/channels in"=w470, "error in"=w471) -> ("task out"=w475:refnum<k21>, "error out"=w474:errorcluster)  [unwired: 12 in]
        n174 = call <vilib>:"DAQmx Clear Task.vi"("task in"=w475, "error in"=w474) -> ("error out"=w476:errorcluster)  [unwired: 13 in]
        n175 = call <vilib>:"Clear Errors.vi"("error in (no error)"=w476) -> ("error out"=w477:errorcluster)  [unwired: 5 in, 1 out]
        n176 = Flush Queue(queue=w469, error in (no error)=w477) -> (error out=w472:errorcluster)  [unwired: 2 out]
      }
      frame "Exit" {
        n177 = Release Queue(queue=w482, error in (no error)=w480) -> (error out=w481:errorcluster)  [unwired: 1 in, 2 out]
      }
    }
    n178 = call "Error Handler - Message Handling Loop.vi"("error in (no error)"=w427, "Message Queue"=w414) -> ("dup error in"=w417:errorcluster)  [unwired: 8 in, 1 out]
  }
  n179 = Unregister For Events(event registration refnum=w30, error in=w28) -> (error out=w31:errorcluster)
  n180 = property on="Data" class="Str"() -> ("Value"=w3:string)  [unwired: 2 in, 2 out]
  n181 = Merge Errors(w31, w33, w24, w17, w13) -> (w11:errorcluster)
  n182 = call "Destroy User Event - Stop.vi"("error in (no error)"=w11, "User Event - Stop"=w18) -> ("error out"=w29:errorcluster)  [unwired: 9 in]
  n183 = call "File Name.vi"("string"=w3) -> ("String"=w4:string)  [unwired: 10 in]
  n184 = Array To Spreadsheet String(array=w9, 3:"%f" ("format string")) -> (spreadsheet string=w5:string)  [unwired: 1 in]
  n185 = disable-structure shown="RUN_TIME_ENGINE==True" {
    disable-tunnel: w29 -> [_ _]
    frame condition #0 (active) {
    }
    frame condition #1 {
      # "Call Quit LabVIEW if running as a built application."
      n186 = Quit LabVIEW() -> ()  [unwired: 1 in]
    }
  }
  n187 = call "Write.vi"("File Name"=w4, "text"=w5) -> ()  [unwired: 9 in, 1 out]
